vi "Get Channel Group Names.vi"(8 "error in":errorcluster, 11 "Document in":refnum<k20>) -> (0 "error out":errorcluster, 2 "Channel Group Details":cluster{"Group Name":string, "Type":string}[](array[cluster]), 3 "Document out":refnum<k20>)   [LabVIEW 2026]
uses:
  Types/NodeFilteringOptions.ctl
  <vilib>/xml/Get Node Text Content (String).vi
  <resource>/objmgr/DOMUserDefRef.rc
  <vilib>/xml/NI_XML.lvlib
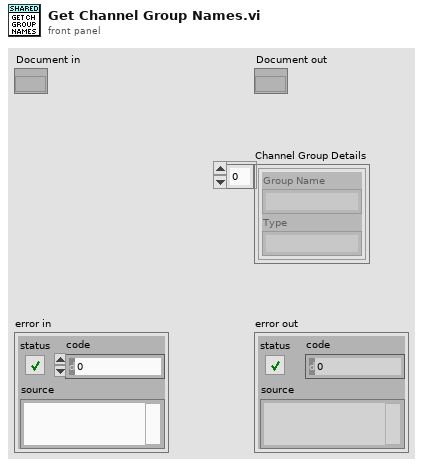
[diagram p1: front panel]
types:
  T1 = typedef "NodeFilteringOptions.ctl" = enum16{"GetCustomDeviceNode", "GetAllChannelNodes", "GetAllSectionNodes", "GetAllWaveformNodes", "GetFirstChannelNode", "GetFirstSectionNode", "GetFirstWaveformNode", "GetSpecificSectionNode", "GetSpecificCustomDeviceNode", "GetSpecificChannelNode", "GetSpecificWaveformNode", "GetMatchedNamedNode", "GetEnumDefinitionsNode", "GetSpecificEnumDefinitionNode", "GetAllEnumDefinitionNodes", "GetDynamicChannelNodes"}
  T2 = cluster{"Attribute Value":string, "node text":string}
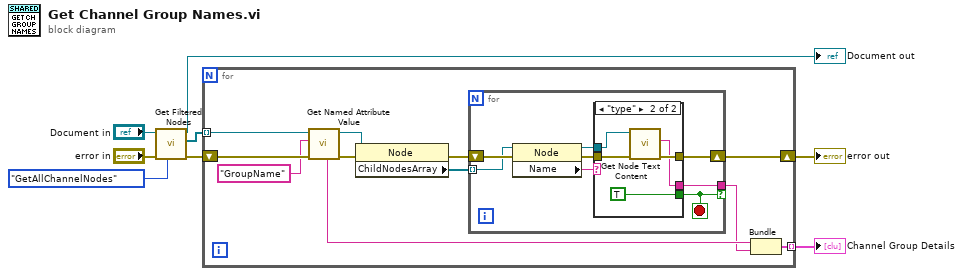
[diagram p0: block diagram]
diagram:
  n1 = call "Get Filtered Nodes.vi"("Node Filtering"=NodeFilteringOptions."GetAllChannelNodes", "error in"="error in", "Document in"="Document in") -> ("error out"=w5:errorcluster, "Filtered Nodes"=w6:refnum<k20>[], "Document out"=→"Document out":refnum<k20>)  [unwired: 4 in, 2 out]
  n2 = for {
    shift-right: [w12] -> w4
    shift-left: w5 -> [w19]
    tunnel: w6 -> [w18] mode=indexing
    tunnel: [w9] -> w3 mode=indexing
    n3 = call "Get Named Attribute Value.vi"("error in"=w19, "Attribute Name"="GroupName", "Node In"=w18) -> ("error out"=w15:errorcluster, "Node Out"=w16:refnum<k20>, "Attribute Value"=w11:string)  [unwired: 5 in, 1 out]
    n4 = property class="Node"(reference=w16, error in=w15) -> (error out=w13:errorcluster, "ChildNodesArray"=w14:refnum<k20>[])  [unwired: 1 out]
    n5 = for {
      tunnel: w14 -> [w21] mode=indexing
      shift-right: [w24] -> w12
      shift-left: w13 -> [w27]
      tunnel: [w23] -> w10 if=w22
      stop <- w22 stop-if-true
      n6 = property class="Node"(reference=w21, error in=w27) -> (reference out=w20:refnum<k20>, error out=w25:errorcluster, "Name"=w26:string)
      n7 = case shown="\"type\"" w26 {
        tunnel: w25 -> [w28 w31]
        tunnel: [w28 w32] -> w24
        tunnel: [_ w29] -> w23
        tunnel: [_ TRUE] -> w22
        tunnel: w20 -> [_ w30]
        frame Default {
        }
        frame "type" {
          n8 = call-poly <vilib>:"Get Node Text Content.vi"("error in (no error)"=w31, "node in"=w30) -> ("error out"=w32:errorcluster, "node text"=w29:string)  [unwired: 7 in, 1 out]
        }
      }
    }
    n9 = Bundle("Attribute Value"=w11, "node text"=w10) -> (w9:T2)  [unwired: 1 in]
  }
  "error out" <- w4
  "Channel Group Details" <- w3
